vi "Is_Dynam_Dispatch.vi"(8 "error in (no error)":errorcluster, 11 "AB_Source_VI in":refnum<class "AB_Source_VI.lvclass">) -> (0 "error out":errorcluster, 2 "dynamicDispatch":bool, 3 "AB_Source_VI out":refnum<class "AB_Source_VI.lvclass">)   [LabVIEW 2020, in "AB_Source_VI.lvclass"]
uses:
  <vilib>/AppBuilder/AB_Classes/Source/VI/AB_Source_VI.lvclass
  <vilib>/AppBuilder/AB_Classes/Source/VI/AB_Source_VI.lvclass/AB_Source_VI.ctl
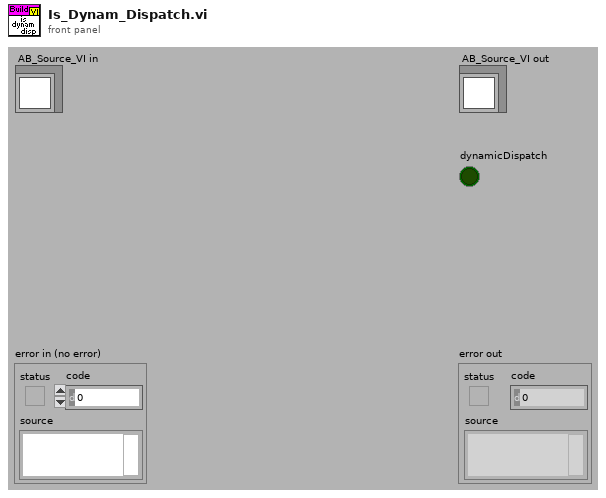
[diagram p1: front panel]
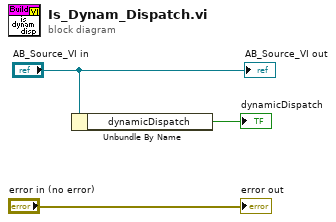
[diagram p0: block diagram]
diagram:
  n1 = Unbundle By Name("AB_Source_VI in") -> ("dynamicDispatch"=→"dynamicDispatch":bool)
  "error out" <- "error in (no error)"
  "AB_Source_VI out" <- "AB_Source_VI in"
